vi "glb_ackTable.vi"() -> ()   [LabVIEW 2014]
panel:
  out "ACK table":bool[](array[boolean])
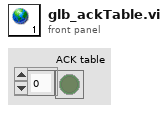
[diagram p1: front panel]
diagram:
